vi "arrayproper.vi"() -> ()   [LabVIEW 2019]
panel:
  out "sum":i16
  in  "String 2":string
  in  "String":string
  out "x = y?":bool[](array[boolean])
  out "deleted portion":dbl[](array[numeric])
  out "array":dbl[](array[numeric])
  in  "length":i32
  out "element":dbl
  in  "index":i32
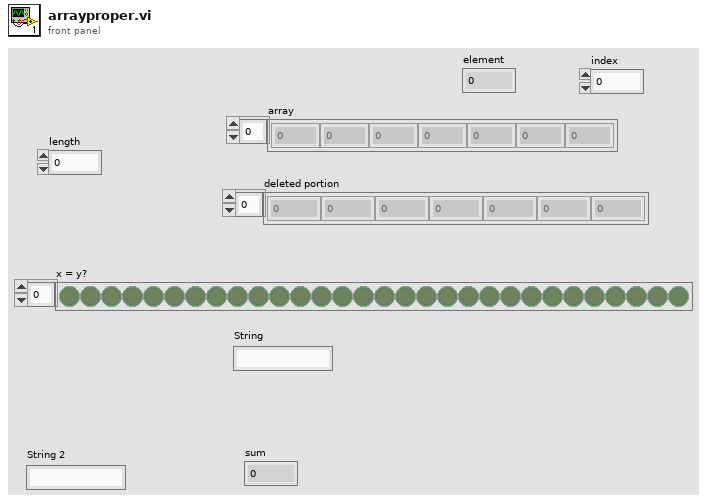
[diagram p1: front panel]
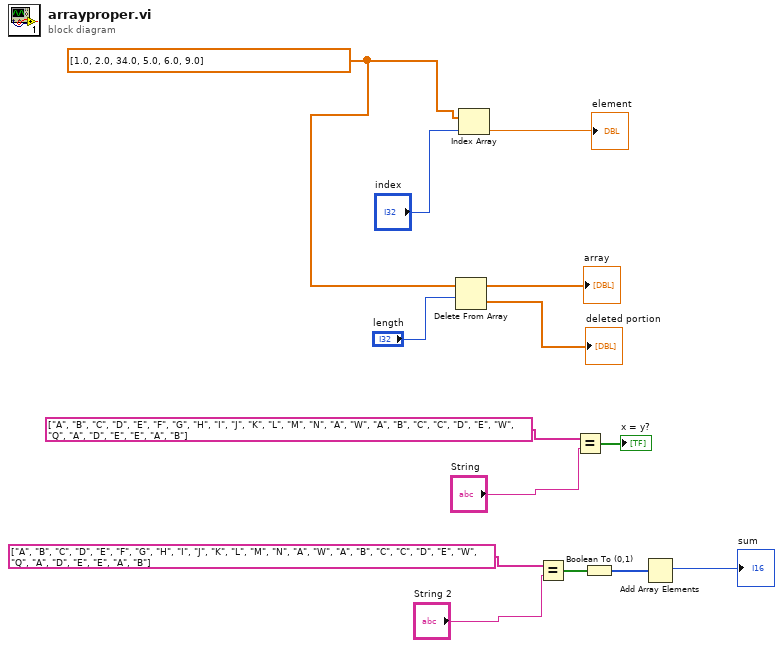
[diagram p0: block diagram]
diagram:
  w12 = dbl[] [1.0, 2.0, 34.0, 5.0, 6.0, 9.0]
  n1 = Delete From Array(array=w12, length="length") -> (deleted portion=→"deleted portion":dbl[], array with subset deleted=→"array":dbl[])  [unwired: 1 in]
  n2 = Index Array(array=w12, index="index") -> (element=→"element":dbl)
  n3 = Equal?(x=string[] ["A", "B", "C", "D", "E", "F", "G", "H", "I", "J", "K", "L", "M", "N", "A", "W", "A", "B", "C", "C", "D", "E", "W", "Q", "A", "D", "E", "E", "A", "B"], y="String 2") -> (x = y?=w3:bool[])
  n4 = Equal?(x=string[] ["A", "B", "C", "D", "E", "F", "G", "H", "I", "J", "K", "L", "M", "N", "A", "W", "A", "B", "C", "C", "D", "E", "W", "Q", "A", "D", "E", "E", "A", "B"], y="String") -> (x = y?=→"x = y?":bool[])
  n5 = Boolean To (0,1)(Boolean=w3) -> (0, 1=w2:i16[])
  n6 = Add Array Elements(numeric array=w2) -> (sum=→"sum":i16)
